vi "get num hydrolysis reactors.vi"(8 "error in (no error)":errorcluster) -> (0 "error out":errorcluster, 3 "function return":i32)   [LabVIEW 2019, in "libSimulationControl.lvlib"]
doc: "int get_num_hydrolysis_reactors();"
uses:
  libSimulationControl.lvlib
  libSimulationControl.so
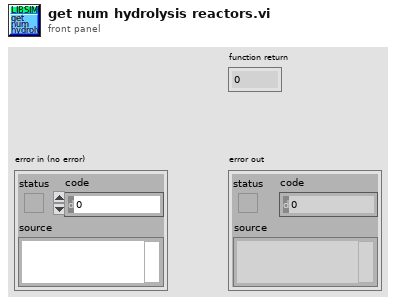
[diagram p1: front panel]
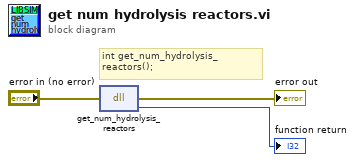
[diagram p0: block diagram]
diagram:
  # "int get_num_hydrolysis_reactors();"
  n1 = dll-call lib="home/paul/Schreibtisch/Biogas_plant_setup/LabView/lib/libSimulationControl/libSimulationControl.*" fn="get_num_hydrolysis_reactors"(error in="error in (no error)") -> (error out=→"error out":errorcluster, →"function return":i32)  [unwired: 2 in, 1 out]
